vi "Disconnect.vi"(8 "error in (no error)":errorcluster, 11 "SimELoad in":refnum<class "SimEload.lvclass">) -> (0 "error out":errorcluster, 3 "SimELoad out":refnum<class "SimEload.lvclass">)   [LabVIEW 2019, in "SimELoad.lvlib" / "SimEload.lvclass"]
uses:
  SimEload.lvclass
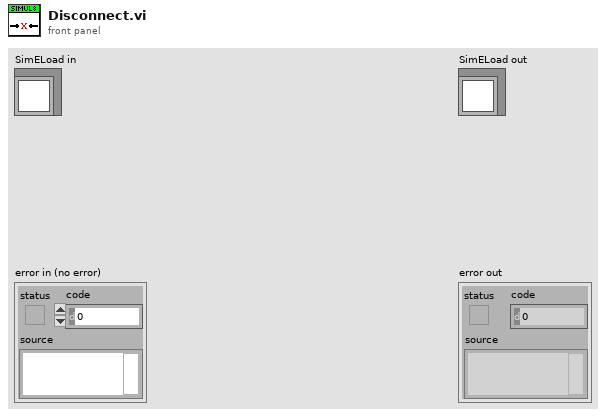
[diagram p1: front panel]
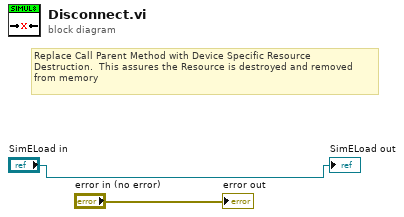
[diagram p0: block diagram]
diagram:
  # "Replace Call Parent Method with Device Specific Resource\nDestruction.  This assures the Resource is destroyed and removed\nfrom memory"
  "error out" <- "error in (no error)"
  "SimELoad out" <- "SimELoad in"
